vi "logging_write.vi"(7 "Add call chain offset\n(No call chain)":i32=-1, 8 "error in":errorcluster caption="error in (no error)", 10 "String to write":string, 11 "VISA resource name":refnum<visa-resource-name>) -> (0 "error out":errorcluster, 3 "VISA resource name out":refnum<visa-resource-name>)   [LabVIEW 2022 SP3, in "hmp4000_rsidr_core.lvlib"]
uses:
  hmp4000_rsidr_core.lvlib
  _type_Logging_Parameter.ctl
  type_Error_Codes.ctl
  Trim Whitespace One-Sided.vi
panel:
  in  "Last Reported Warning":string
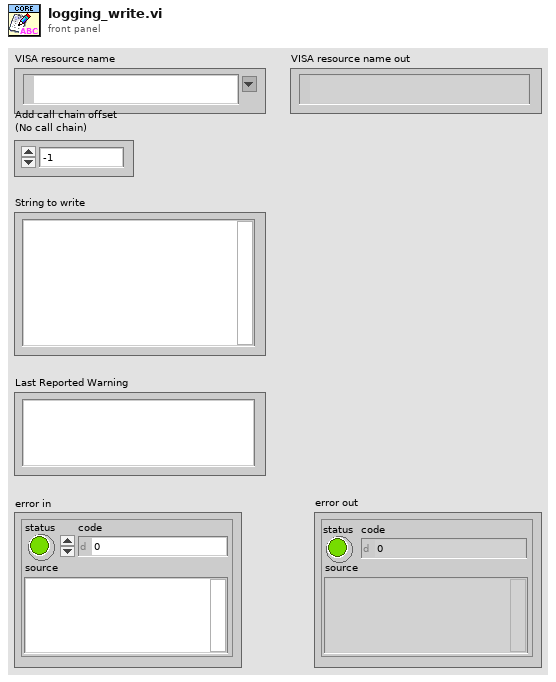
[diagram p1: front panel]
types:
  T1 = typedef "hmp4000_rsidr_core.lvlib/type_Session_Data.ctl" = cluster{"IDN string":string, "Instrument FW":string, "Instr type":string, "Instr type for err. msg.":string, "Installed Options":string[], "Ignore Error Messages":string, "Logging params":variant, "OPC Timeout":i32, "VISA Timeout":i32, "STB Poll VISA Timeout":i32, "Additional Flags":i32, "Wait Before Read":i32, "Wait Before Write":i32, "Option String Flags":i32, "IO Segment Size":i64, "VISA Access Mode":T2, "Interface Type":T3, "OPC Wait Mode":T4, "Bin Float Number  Format":T5, "Bin Integer Number Format":T6, "Simulate":bool, "VXIcapable":bool, "Duplicate Session":bool, "Add LF to Write":bool, "Logging":bool, "Fast Sweep":bool, "Query Instrument Status":bool, "Check Range":bool, "Check Options":bool}
  T2 = typedef "hmp4000_rsidr_core.lvlib/type_VisaAccessMode.ctl" = u16
  T3 = typedef "hmp4000_rsidr_core.lvlib/type_InterfaceType.ctl" = enum16{"Unknown", "GPIB", "VXI", "GPIB_VXI", "ASRL", "PXI", "TCPIP", "USB", "SOCKET"}
  T4 = typedef "hmp4000_rsidr_core.lvlib/type_OPC_Wait_Mode.ctl" = enum16{"STBpolling", "STBpollingSlow", "STBpollingSuperSlow", "ServiceRequest", "OPCquery"}
  T5 = typedef "hmp4000_rsidr_core.lvlib/type_Binary_Float_Number_Format.ctl" = enum16{"Float_4_Bytes_Swapped", "Float_4_Bytes", "Double_8_Bytes_Swapped", "Double_8_Bytes"}
  T6 = typedef "hmp4000_rsidr_core.lvlib/type_Binary_Integer_Number_Format.ctl" = enum16{"Int32_4_Bytes_Swapped", "Int32_4 Bytes", "Int16_2_Bytes_Swapped", "Int16_2_Bytes"}
  T7 = typedef "hmp4000_rsidr_core.lvlib/_type_Logging_Parameter.ctl" = enum16{"Type (String)", "SessionAlias(String)", "FormatString (String)", "UDPconectionID (I32)", "UDPlocalPort (I32)", "UDPremotePort (I32)", "UDPremoteHost (String)", "FILEmode (I32)", "FILEpath (String)", "FILEopenID (I32)", "DataMaxLogLen (I32)"}
  T8 = typedef "hmp4000_rsidr_core.lvlib/type_Error_Codes.ctl" = enum16{"No_error", "VISA_err_ResourceNotFound", "VISA_err_Timeout", "VISA_warn_MoreDataAvailable", "RS_err_MissingCallback", "RS_err_InvalidAttribute", "RS_err_InvalidValue", "RS_err_UnknownResource", "RS_err_AlreadyInitialized", "RS_err_InstrumentStatus", "RS_err_BadRepCapName", "RS_err_TypesMismatch", "RS_err_ValueNotSupported", "RS_err_InvalidRngTable", "RS_err_IDqueryFail", "RS_err_UnexpResponse", "VISA_warn_ConfigNotLoaded", "RS_err_AttributeNotReadable", "RS_err_AttributeNotWritable", "RS_err_InstrumentType", "RS_err_InstrumentOption", "VISA_err_InvalidSize", "RS_err_ReliabilityIndicator", "VISA_warn_UnknownStatus", "VISA_warn_TermCharRead", "VISA_err_IO_error", "RS_err_FunctionNotSupported", "VISA_warn_QueueEmpty"}
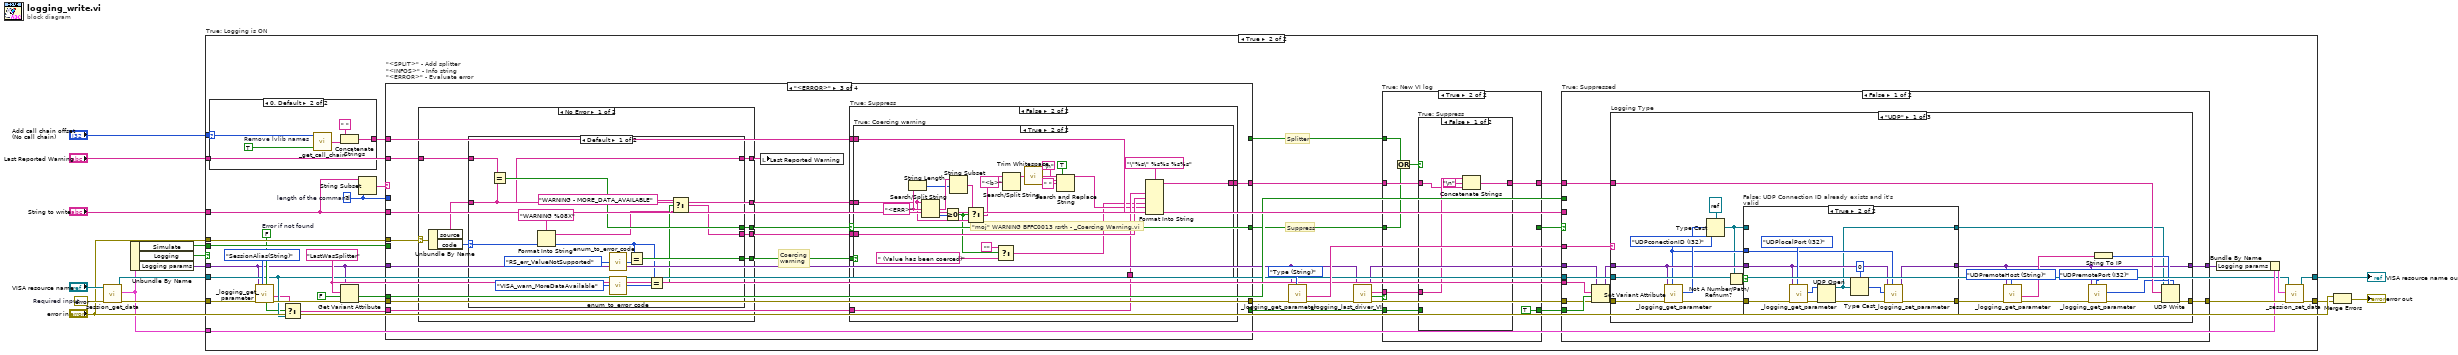
[diagram p0: block diagram]
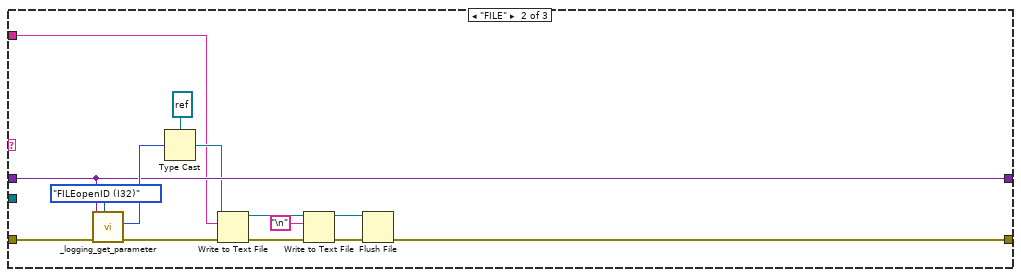
[diagram p6: hidden frame]
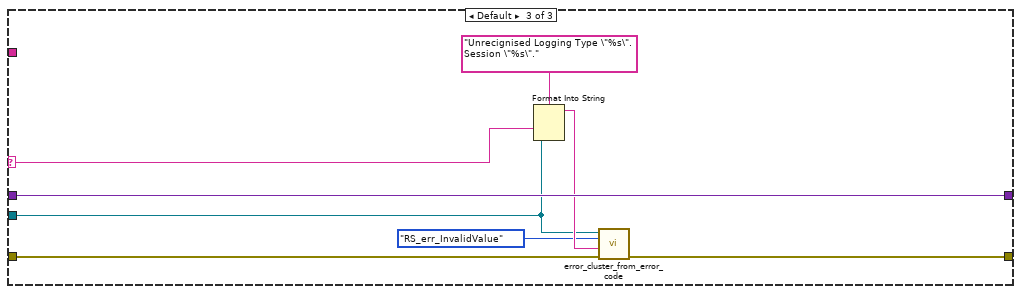
[diagram p7: hidden frame]
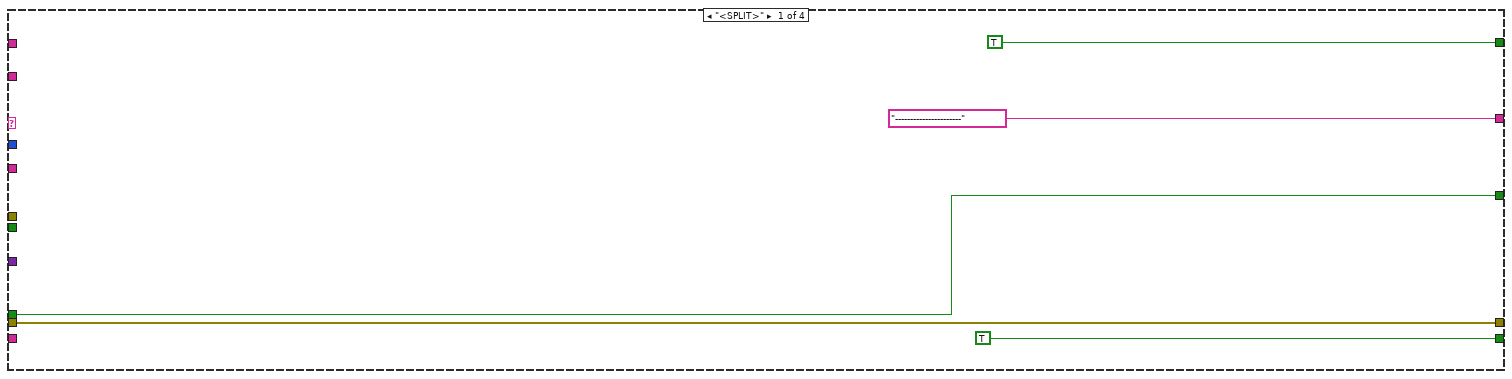
[diagram p10: hidden frame]
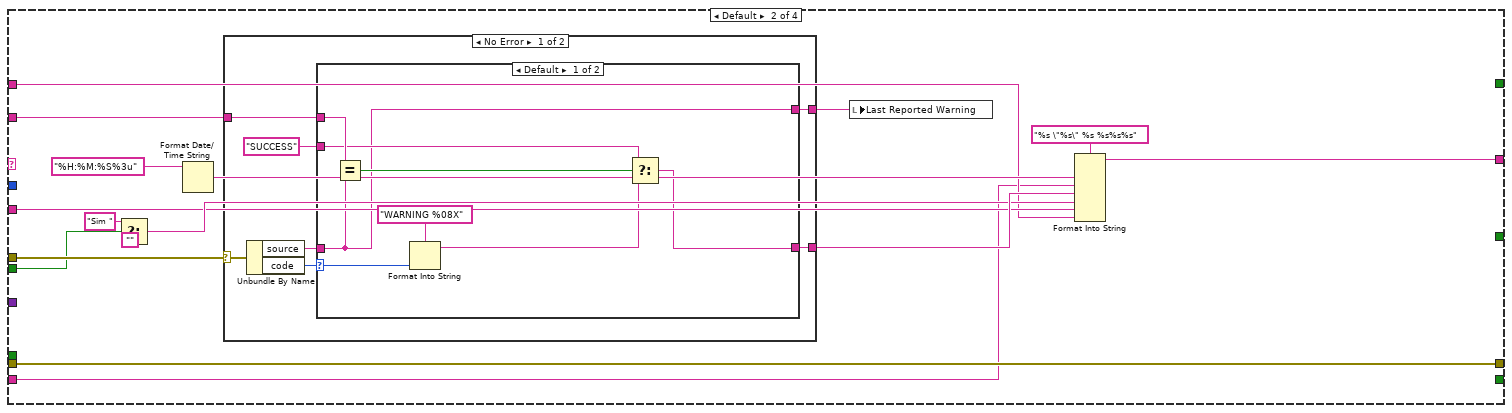
[diagram p11: hidden frame]
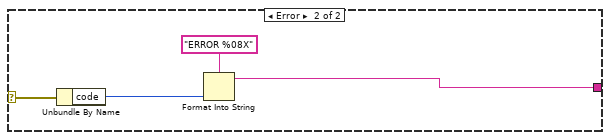
[diagram p13: hidden frame]
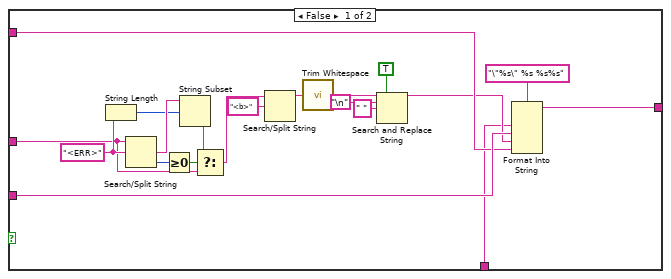
[diagram p15: hidden frame]
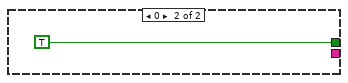
[diagram p16: hidden frame]
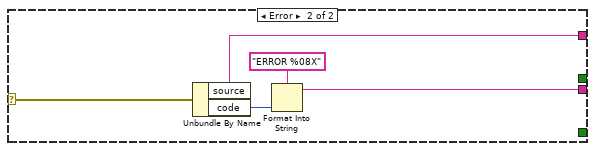
[diagram p17: hidden frame]
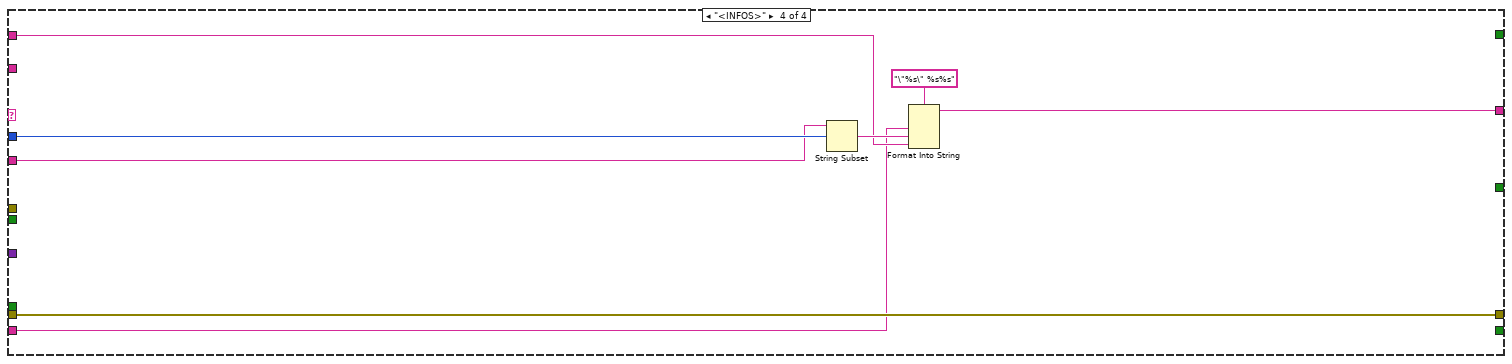
[diagram p18: hidden frame]
diagram:
  w10 = errorcluster {"status"=FALSE, "code"=0, "source"=""}  # Required input
  n1 = call "session_get_data.vi"("error in"=w10, "VISA resource name"="VISA resource name") -> ("error out"=w13:errorcluster, "Session User Data out"=w4:T1, "VISA resource name out"=w5:refnum<visa-resource-name>)  [unwired: 6 in, 1 out]
  n2 = Unbundle By Name(w4) -> ("Simulate"=w6:bool, "Logging"=w11:bool, "Logging params"=w12:variant)
  n3 = case "True: Logging is ON" shown="True" w11 {
    tunnel: w13 -> [w17 w40]
    tunnel: [w17 w51] -> w8
    tunnel: w12 -> [_ w30]
    tunnel: w5 -> [w16 w36]
    tunnel: "String to write" -> [_ w42]
    tunnel: "error in" -> [_ w59]
    tunnel: w6 -> [_ w58]
    tunnel: w4 -> [_ w50]
    tunnel: [w16 w47] -> w3
    tunnel: "Add call chain offset\n(No call chain)" -> [_ w19]
    tunnel: "Last Reported Warning" -> [_ w18]
    frame False {
    }
    frame True {
      w37 = FALSE  # Error if not found
      w44 = "LastWasSplitter" ("name")
      w56 = 7  # length of the command
      # "Splitter"
      # "Suppress"
      n4 = case shown="0, Default" w19 {
        selector: w19 -> [_ w150]
        tunnel: [_ w147] -> w55
        frame -1 {
        }
        frame 0, Default {
          w149 = TRUE  # Remove lvlib names
          n5 = call "_get_call_chain.vi"("Remove lvlib names (F)"=w149, "Cut first x elements\nfrom Error Chain (0)"=w150) -> ("Call chain out in spreadsheet string"=w148:string)  [unwired: 1 in, 2 out]
          n6 = Concatenate Strings(" ", w148) -> (w147:string)
        }
      }
      n7 = call "_logging_get_parameter.vi"("Error if not found (T)"=w37, "Logging Parameter"=_type_Logging_Parameter."SessionAlias(String)", "error in"=w40, "Logging params in"=w30) -> ("error out"=w38:errorcluster, "String parameter out"=w34:string, "Found"=w35:bool)  [unwired: 3 in, 2 out]
      n8 = Select(t=w34, s=w35, f=w36) -> (s? t:f=w33:string)
      n9 = Get Variant Attribute(Variant=w30, name=w44, default value (empty Variant)=FALSE, error in=w38) -> (value=w41:bool, error out=w53:errorcluster)  [unwired: 2 out]
      n10 = String Subset(string=w42, length (rest)=w56) -> (substring=w43:string)  [unwired: 1 in]
      n11 = case "\"<SPLIT>\" - Add splitter\n\"<INFOS>\" - Info string\n\"<ERROR>\" - Evaluate error" shown="\"<ERROR>\"" w43 {
        tunnel: ["----------------------" w168 w202 w282] -> w24
        tunnel: w59 -> [_ w167 w201 _]
        tunnel: w58 -> [_ w166 _ _]
        tunnel: w53 -> [w155 w159 w199 w285]
        tunnel: w30 -> [_ _ _ _]
        tunnel: [w155 w159 w199 w285] -> w45
        tunnel: w42 -> [_ w161 _ w286]
        tunnel: w56 -> [_ _ _ w287]
        tunnel: w41 -> [w153 _ _ _]
        tunnel: [w153 _ w195 _] -> w26
        tunnel: w55 -> [_ w160 w198 w281]
        tunnel: [TRUE _ _ _] -> w21
        tunnel: w33 -> [_ w158 w196 w280]
        tunnel: [TRUE _ _ _] -> w27
        tunnel: w18 -> [_ w157 w193 _]
        frame "<SPLIT>" {
        }
        frame Default {
          n12 = Select(t="Sim " ("time format string (%c)"), s=w166, f="" ("Empty String Constant")) -> (s? t:f=w162:string)
          n13 = Format Date/Time String(time format string (%c)="%H:%M:%S%3u") -> (date/time string=w169:string)  [unwired: 2 in]
          n14 = case shown="No Error" w167 {
            selector: w167 -> [w178 w191]
            tunnel: [w176 w189] -> w163
            tunnel: w157 -> [w175 _]
            tunnel: [w172 _] -> w156
            frame No Error {
              n15 = Unbundle By Name(w178) -> ("source"=w174:string, "code"=w177:i32)
              n16 = case shown="Default" w177 {
                selector: w177 -> [w185 _]
                tunnel: [w182 w187] -> w176
                tunnel: w175 -> [w184 _]
                tunnel: w174 -> [w179 _]
                tunnel: "SUCCESS" -> [w180 w187]
                tunnel: [w179 _] -> w172
                frame Default {
                  n17 = Equal?(x=w184, y=w179) -> (x = y?=w183:bool)
                  n18 = Format Into String(format string="WARNING %08X", w185) -> (resulting string=w181:string)  [unwired: 2 in, 1 out]
                  n19 = Select(t=w180, s=w183, f=w181) -> (s? t:f=w182:string)
                }
                frame 0 {
                }
              }
            }
            frame Error {
              n20 = Unbundle By Name(w191) -> ("code"=w188:i32)
              n21 = Format Into String(format string="ERROR %08X", w188) -> (resulting string=w189:string)  [unwired: 2 in, 1 out]
            }
          }
          n22 = local write "Last Reported Warning"(w156) -> ()
          n23 = Format Into String(format string="%s \"%s\" %s %s%s%s", w169, w158, w163, w162, w161, w160) -> (resulting string=w168:string)  [unwired: 2 in, 1 out]
        }
        frame "<ERROR>" {
          # "Coercing\nwarning"
          n24 = case shown="No Error" w201 {
            selector: w201 -> [w259 w279]
            tunnel: [w258 w277] -> w200
            tunnel: [w253 w276] -> w197
            tunnel: [w257 _] -> w195
            tunnel: [w255 _] -> w194
            tunnel: w193 -> [w254 _]
            tunnel: [w252 _] -> w192
            frame No Error {
              n25 = Unbundle By Name(w259) -> ("source"=w253:string, "code"=w256:i32)
              n26 = case shown="Default" w256 {
                selector: w256 -> [w264 _]
                tunnel: [w260 _] -> w258
                tunnel: [w268 TRUE] -> w257
                tunnel: [w270 _] -> w255
                tunnel: w254 -> [w269 _]
                tunnel: w253 -> [w267 _]
                tunnel: [w267 _] -> w252
                frame Default {
                  n27 = Equal?(x=w269, y=w267) -> (x = y?=w268:bool)
                  n28 = Format Into String(format string="WARNING %08X", w264) -> (resulting string=w262:string)  [unwired: 2 in, 1 out]
                  n29 = call "enum_to_error_code.vi"("Error Enum in"=type_Error_Codes."RS_err_ValueNotSupported") -> ("error code out"=w271:i32)  [unwired: 4 in]
                  n30 = call "enum_to_error_code.vi"("Error Enum in"=type_Error_Codes."VISA_warn_MoreDataAvailable") -> ("error code out"=w265:i32)  [unwired: 4 in]
                  n31 = Equal?(x=w264, y=w271) -> (x = y?=w270:bool)
                  n32 = Equal?(x=w264, y=w265) -> (x = y?=w263:bool)
                  n33 = Select(t="WARNING - MORE_DATA_AVAILABLE" ("format string"), s=w263, f=w262) -> (s? t:f=w260:string)
                }
                frame 0 {
                }
              }
            }
            frame Error {
              n34 = Unbundle By Name(w279) -> ("source"=w276:string, "code"=w275:i32)
              n35 = Format Into String(format string="ERROR %08X", w275) -> (resulting string=w277:string)  [unwired: 2 in, 1 out]
            }
          }
          n36 = local write "Last Reported Warning"(w192) -> ()
          n37 = case "True: Suppress" shown="False" w195 {
            tunnel: [_ w208] -> w202
            tunnel: w200 -> [_ w207]
            tunnel: w198 -> [_ w206]
            tunnel: w197 -> [_ w205]
            tunnel: w196 -> [_ w204]
            tunnel: w194 -> [_ w203]
            frame True {
            }
            frame False {
              n38 = case "True: Coercing warning" shown="True" w203 {
                tunnel: [w227 w250] -> w208
                tunnel: w207 -> [w226 w249]
                tunnel: w206 -> [w225 w231]
                tunnel: w205 -> [w218 w244]
                tunnel: w204 -> [w209 w238]
                frame False {
                  w221 = "<ERR>" ("search string/char (-)")
                  n39 = String Length(string=w221) -> (length=w220:i32)
                  n40 = Search/Split String(string=w218, search string/char (-)=w221) -> (match + rest of string=w222:string, offset of match=w224:i32)  [unwired: 1 in, 1 out]
                  n41 = Greater Or Equal To 0?(x=w224) -> (x >= 0?=w223:bool)
                  n42 = String Subset(string=w222, offset (0)=w220) -> (substring=w219:string)  [unwired: 1 in]
                  n43 = Select(t=w219, s=w223, f=w218) -> (s? t:f=w217:string)
                  n44 = Search/Split String(string=w217, search string/char (-)="<b>") -> (substring before match=w215:string)  [unwired: 1 in, 2 out]
                  n45 = call "Trim Whitespace.vi"("string"=w215) -> ("trimmed string"=w213:string)  [unwired: 1 in]
                  n46 = Search and Replace String(replace all?=TRUE ("replace all? (F)"), input string=w213, search string="\n" ("Line Feed Constant"), replace string=" " ("replace string (\"\")")) -> (result string=w210:string)  [unwired: 4 in, 3 out]
                  n47 = Format Into String(format string="\"%s\" %s %s%s", w209, w226, w210, w225) -> (resulting string=w227:string)  [unwired: 2 in, 1 out]
                }
                frame True {
                  w246 = "<ERR>" ("search string/char (-)")
                  # "\"moj\" WARNING BFFC0013 rsrth - _Coercing Warning.vi"
                  n48 = String Length(string=w246) -> (length=w245:i32)
                  n49 = Search/Split String(string=w244, search string/char (-)=w246) -> (match + rest of string=w247:string, offset of match=w248:i32)  [unwired: 1 in, 1 out]
                  n50 = Greater Or Equal To 0?(x=w248) -> (x >= 0?=w234:bool)
                  n51 = String Subset(string=w247, offset (0)=w245) -> (substring=w235:string)  [unwired: 1 in]
                  n52 = Select(t=w235, s=w234, f=w244) -> (s? t:f=w237:string)
                  n53 = Select(t="" ("Empty String Constant"), s=w234, f=" (Value has been coerced)" ("search string/char (-)")) -> (s? t:f=w229:string)
                  n54 = Search/Split String(string=w237, search string/char (-)="<b>") -> (substring before match=w242:string)  [unwired: 1 in, 2 out]
                  n55 = call "Trim Whitespace.vi"("string"=w242) -> ("trimmed string"=w240:string)  [unwired: 1 in]
                  n56 = Search and Replace String(replace all?=TRUE ("replace all? (F)"), input string=w240, search string="\n" ("Line Feed Constant"), replace string=" " ("replace string (\"\")")) -> (result string=w230:string)  [unwired: 4 in, 3 out]
                  n57 = Format Into String(format string="\"%s\" %s%s %s%s", w238, w249, w229, w230, w231) -> (resulting string=w250:string)  [unwired: 2 in, 1 out]
                }
              }
            }
          }
        }
        frame "<INFOS>" {
          n58 = String Subset(string=w286, offset (0)=w287) -> (substring=w283:string)  [unwired: 1 in]
          n59 = Format Into String(format string="\"%s\" %s%s", w280, w283, w281) -> (resulting string=w282:string)  [unwired: 2 in, 1 out]
        }
      }
      n60 = call "_logging_get_parameter.vi"("Logging Parameter"=_type_Logging_Parameter."Type (String)", "error in"=w45, "Logging params in"=w30) -> ("error out"=w32:errorcluster, "String parameter out"=w46:string)  [unwired: 4 in, 3 out]
      n61 = call "_logging_last_driver_VI.vi"("error in"=w32, "Logging params in"=w30) -> ("error out"=w31:errorcluster, "VI changed"=w28:bool, "New VI string"=w22:string, "Logging params out"=w29:variant)  [unwired: 6 in]
      n62 = case "True: New VI log" shown="True" w28 {
        tunnel: w27 -> [_ w66]
        tunnel: w26 -> [w62 w67]
        tunnel: [w62 _] -> w25
        tunnel: w24 -> [w61 w69]
        tunnel: [w61 w70] -> w23
        tunnel: w22 -> [_ w68]
        tunnel: w21 -> [w60 w64]
        tunnel: [w60 TRUE] -> w20
        frame False {
        }
        frame True {
          n63 = Or(x=w66, y=w67) -> (x .or. y?=w65:bool)
          n64 = case "True: Suppress" shown="False" w65 {
            tunnel: [w73 w75] -> w70
            tunnel: w69 -> [w71 _]
            tunnel: w68 -> [w74 w75]
            tunnel: w64 -> [_ _]
            frame False {
              n65 = Concatenate Strings(w74, "\n" ("Line Feed Constant"), w71) -> (w73:string)
            }
            frame True {
            }
          }
        }
      }
      n66 = case "True: Suppressed" shown="False" w25 {
        tunnel: w23 -> [w86 _]
        tunnel: w31 -> [w78 w145]
        tunnel: w29 -> [w81 w144]
        tunnel: [w85 w145] -> w52
        tunnel: w36 -> [w84 _]
        tunnel: [w83 w144] -> w48
        tunnel: w46 -> [w82 _]
        tunnel: w20 -> [w80 _]
        tunnel: w44 -> [w79 _]
        tunnel: w42 -> [_ _]
        tunnel: w41 -> [_ _]
        frame False {
          n67 = Set Variant Attribute(Variant=w81, name=w79, value=w80, error in=w78) -> (Variant out=w77:variant, error out=w76:errorcluster)  [unwired: 1 out]
          n68 = case "Logging Type" shown="\"UDP\"" w82 {
            selector: w82 -> [_ _ w143]
            tunnel: w76 -> [w103 w135 w141]
            tunnel: [w105 w127 w140] -> w85
            tunnel: w84 -> [_ _ w136]
            tunnel: w86 -> [w104 w129 _]
            tunnel: w77 -> [w92 w132 w139]
            tunnel: [w90 w132 w139] -> w83
            frame "UDP" {
              w91 = _type_Logging_Parameter."UDPconectionID (I32)" ("Logging Parameter")
              n69 = call "_logging_get_parameter.vi"("Logging Parameter"=w91, "error in"=w103, "Logging params in"=w92) -> ("error out"=w94:errorcluster, "Int32 parameter out"=w96:i32)  [unwired: 4 in, 3 out]
              n70 = Type Cast(type=refnum<k16> refnum ("connection ID"), x=w96) -> (*(type *) &x=w88:refnum<k16>)
              n71 = Not A Number/Path/Refnum?(number/path/refnum=w88) -> (NaN/Path/Refnum?=w89:bool)
              n72 = case "False: UDP Connection ID already exists and it's valid" shown="True" w89 {
                tunnel: w94 -> [w109 w121]
                tunnel: [w109 w116] -> w93
                tunnel: w92 -> [w108 w115]
                tunnel: w91 -> [_ w114]
                tunnel: [w108 w111] -> w90
                tunnel: w88 -> [w107 _]
                tunnel: [w107 w110] -> w87
                frame False {
                }
                frame True {
                  n73 = call "_logging_get_parameter.vi"("Logging Parameter"=_type_Logging_Parameter."UDPlocalPort (I32)", "error in"=w121, "Logging params in"=w115) -> ("error out"=w120:errorcluster, "Int32 parameter out"=w118:i32)  [unwired: 4 in, 3 out]
                  n74 = UDP Open(8:w120, 11:w118) -> (port=w110:refnum<k16>, 0:w117:errorcluster)  [unwired: 1 in, 3 out]
                  n75 = Type Cast(type=0, x=w110) -> (*(type *) &x=w112:i32)
                  n76 = call "_logging_set_parameter.vi"("Logging Parameter"=w114, "error in"=w117, "Int32 parameter (0)"=w112, "Logging params in"=w115) -> ("error out"=w116:errorcluster, "Logging params out"=w111:variant)  [unwired: 6 in]
                }
              }
              n77 = call "_logging_get_parameter.vi"("Logging Parameter"=_type_Logging_Parameter."UDPremoteHost (String)", "error in"=w93, "Logging params in"=w90) -> ("error out"=w99:errorcluster, "String parameter out"=w95:string)  [unwired: 4 in, 3 out]
              n78 = call "_logging_get_parameter.vi"("Logging Parameter"=_type_Logging_Parameter."UDPremotePort (I32)", "error in"=w99, "Logging params in"=w90) -> ("error out"=w98:errorcluster, "Int32 parameter out"=w100:i32)  [unwired: 4 in, 3 out]
              n79 = String To IP(1:w95) -> (0:w106:u32)
              n80 = UDP Write(address=w106, port or service name=w100, connection ID=w87, data in=w104, 8:w98) -> (error out=w105:errorcluster)  [unwired: 2 out]
            }
            frame "FILE" {
              n81 = call "_logging_get_parameter.vi"("Logging Parameter"=_type_Logging_Parameter."FILEopenID (I32)", "error in"=w135, "Logging params in"=w132) -> ("error out"=w128:errorcluster, "Int32 parameter out"=w133:i32)  [unwired: 4 in, 3 out]
              n82 = Type Cast(type=refnum<file> refnum ("refnum out"), x=w133) -> (*(type *) &x=w130:refnum<file>)
              n83 = Write to Text File(file (use dialog)=w130, text=w129, error in=w128) -> (refnum out=w124:refnum<file>, error out=w126:errorcluster)  [unwired: 1 in, 1 out]
              n84 = Write to Text File(file (use dialog)=w124, text="\n" ("Line Feed Constant"), error in=w126) -> (refnum out=w123:refnum<file>, error out=w125:errorcluster)  [unwired: 1 in, 1 out]
              n85 = Flush File(refnum=w123, error in=w125) -> (error out=w127:errorcluster)  [unwired: 1 out]
            }
            frame Default {
              n86 = Format Into String(format string="Unrecignised Logging Type \"%s\". Session \"%s\".", w143, w136) -> (resulting string=w138:string)  [unwired: 2 in, 1 out]
              n87 = call "error_cluster_from_error_code.vi"("error in"=w141, "Error Message (\"\")"=w138, "Error Enum in"=type_Error_Codes."RS_err_InvalidValue", "VISA resource name"=w136) -> ("error out"=w140:errorcluster)  [unwired: 6 in, 1 out]
            }
          }
        }
        frame True {
        }
      }
      n88 = Bundle By Name(cluster=w50, "Logging params"=w48) -> (w49:T1)
      n89 = call "_session_set_data.vi"("error in"=w52, "Session User Data in"=w49, "VISA resource name"=w36) -> ("error out"=w51:errorcluster, "VISA resource name out"=w47:refnum<visa-resource-name>)  [unwired: 7 in]
    }
  }
  "VISA resource name out" <- w3
  n90 = Merge Errors("error in", w8) -> (→"error out":errorcluster)
